vi "V7310.Example.GetJobs.vi"() -> ()   [LabVIEW 2016]
uses:
  LowLevel/V7310.Job.Variable.ctl
panel:
  out "error IO":errorcluster
  out "size":i32
  out "idx":i32
  out "Array 2":errorcluster[](array[cluster])
  out "Array":cluster{string, "VarNames":T1[]}[](array[cluster])
  out "size(s)":i32
  out "Jobs":string[](array[string])
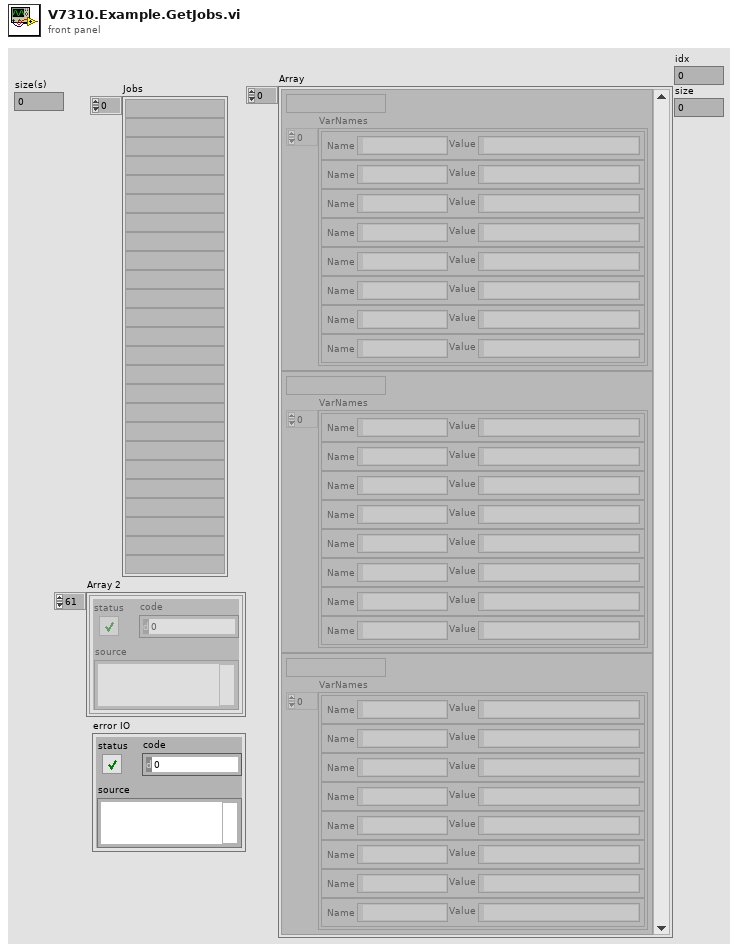
[diagram p1: front panel]
types:
  T1 = typedef "V7310.Job.Variable.ctl" = cluster{"Name":string, "Value":string}
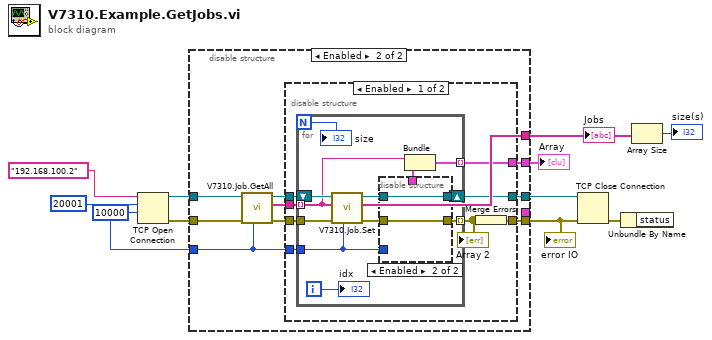
[diagram p0: block diagram]
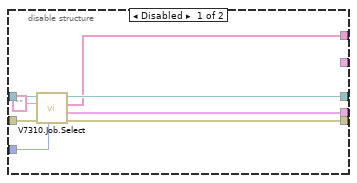
[diagram p2: hidden frame]
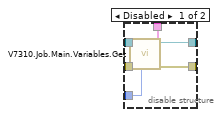
[diagram p3: hidden frame]
diagram:
  w4 = 10000 ("timeout ms (60000)")
  n1 = TCP Open Connection(address="192.168.100.2", remote port or service name=u16 20001, timeout ms (60000)=w4) -> (connection ID=w7:refnum<k5>, error out=w6:errorcluster)  [unwired: 2 in]
  n2 = disable-structure shown="Enabled" {
    disable-tunnel: [w19 w23] -> w9
    disable-tunnel: [w18 w22] -> w8
    disable-tunnel: w7 -> [w17 w27]
    disable-tunnel: w6 -> [w16 w28]
    disable-tunnel: [w15 w26] -> w3
    disable-tunnel: [w14 _] -> _
    disable-tunnel: w4 -> [w13 w20]
    disable-tunnel: [_ w21] -> w1
    frame Disabled {
      n3 = call "V7310.Job.Select.vi"("timeout ms (5000)"=w13, "error in"=w16, "Job"="", "Connection in"=w17) -> ("error out"=w18:errorcluster, "VarNames"=w14:T1[], "Jobs"=w15:string[], "Connection out"=w19:refnum<k5>)  [unwired: 3 in, 1 out]
    }
    frame Enabled {
      n4 = call "V7310.Job.GetAll.vi"("timeout ms (5000)"=w20, "error in"=w28, "Connection in"=w27) -> ("error out"=w25:errorcluster, "Jobs"=w26:string[], "Connection out"=w24:refnum<k5>)  [unwired: 6 in]
      n5 = disable-structure shown="Enabled" {
        disable-tunnel: w26 -> [w36 _]
        disable-tunnel: w25 -> [w35 w58]
        disable-tunnel: w24 -> [w34 w57]
        disable-tunnel: [w33 w57] -> w23
        disable-tunnel: [w31 w58] -> w22
        disable-tunnel: [w30 _] -> w21
        disable-tunnel: w20 -> [w29 _]
        frame Enabled {
          n6 = for {
            N -> [w38]
            tunnel: w36 -> [w41] mode=indexing
            tunnel: w35 -> [w46]
            tunnel: [w42] -> w32 mode=indexing
            shift-right: [w43] -> w33
            shift-left: w34 -> [w45]
            tunnel: [w40] -> w30 mode=indexing
            tunnel: w29 -> [w37]
            i -> [w39]
            n7 = call "V7310.Job.Set.vi"("timeout ms (5000)"=w37, "error in"=w46, "Job"=w41, "Connection in"=w45) -> ("error out"=w48:errorcluster, "Connection out"=w47:refnum<k5>)  [unwired: 6 in]
            n8 = disable-structure shown="Enabled" {
              disable-tunnel: w48 -> [w54 w56]
              disable-tunnel: w47 -> [w53 w55]
              disable-tunnel: [w52 _] -> w44
              disable-tunnel: [w51 w55] -> w43
              disable-tunnel: [w50 w56] -> w42
              disable-tunnel: w37 -> [w49 _]
              frame Disabled {
                n9 = call "V7310.Job.Main.Variables.Get.vi"("timeout ms (5000)"=w49, "error in"=w54, "Connection in"=w53) -> ("error out"=w50:errorcluster, "VarNames"=w52:T1[], "Connection out"=w51:refnum<k5>)  [unwired: 6 in]
              }
              frame Enabled {
              }
            }
            n10 = Bundle(w41, "VarNames"=w44) -> (w40:cluster{string, "VarNames":T1[]})  [unwired: 1 in]
            "idx" <- w39
            "size" <- w38
          }
          "Array 2" <- w32
          n11 = Merge Errors(w32) -> (w31:errorcluster)
        }
        frame Disabled {
        }
      }
    }
  }
  "Jobs" <- w3
  "Array" <- w1
  "error IO" <- w8
  n12 = TCP Close Connection(connection ID=w9, error in (no error)=w8) -> (error out=w10:errorcluster)  [unwired: 1 in, 1 out]
  n13 = Unbundle By Name(w10) -> ()  [unwired: 1 out]
  n14 = Array Size(array=w3) -> (size(s)=→"size(s)":i32)
